vi "Calibrate_Axis_Sub.vi"(4 "Camera":T2="Pencilcam", 5 "Min Position":dbl=-1100.0, 6 "Position of Strip Centre":dbl=50.0, 7 "Max Position":dbl=1000.0, 8 "Time String":string, 9 "Axis to Calibrate":enum16{"X Axis", "Y Axis"}(ring), 10 "Datum Position":sgl[](array[numeric])=[0.0, 0.0, 50.0] format="%#.2f", 11 "Traverse Name":string="EnFlo_Stack") -> (0 "Status":T1, 1 "Correction Folder":path)   [LabVIEW 2015]
uses:
  Camera Server/Camera enum/Camera enum.ctl
  Multi_Run_Status.ctl
  Traverse_cluster.ctl
  Spacing.ctl
  Controls/Multi_run_mode.ctl
  Utilities/Image acquisition and processing/Feature detection/Typedefs/Top level controls.ctl
  Utilities/Image acquisition and processing/Feature detection/Typedefs/Theta range.ctl
  Utilities/Image acquisition and processing/Feature detection/Typedefs/Txy range.ctl
  Utilities/Image acquisition and processing/Feature detection/Typedefs/ROI bounds.ctl
  Camera Server/Camera enum/Camera resolution.ctl
  Controls/Tunnel_Coordinates.ctl
  Globals/Constants_global.vi
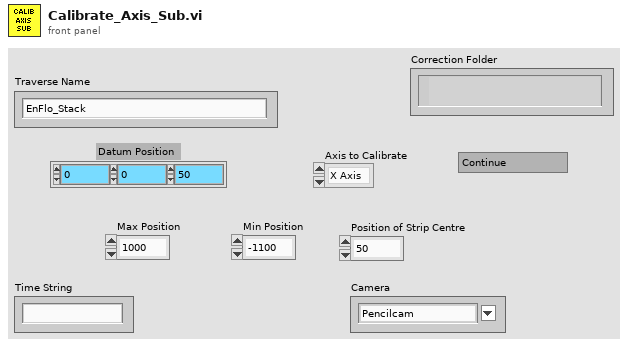
[diagram p1: front panel]
types:
  T1 = typedef "Multi_Run_Status.ctl" = enum16{"Continue", "Jump to Next Point", "Jump to Next Row", "Jump To Fall Back", "Terminate Run"}
  T2 = typedef "Camera enum.ctl" = string
  T3 = typedef "Traverse_cluster.ctl" = cluster{"Start X":sgl, "Start Y":sgl, "Start Z":sgl, "End X":sgl, "End Y":sgl, "End Z":sgl, "No. of pts.":i32, "Spacing":T4, "Filename":path, "Tunnel Speed":dbl, "Averaging time (min)":dbl, "Extra Commands":string, "Carrier_1 Q (l/min)":dbl, "Carrier_2 Q (l/min)":dbl, "Trace Gas Concentration (%)":dbl, "Specific Arguments":string, "Comments":string, "Row No":i32, "Row Type Selector":T5, "Completion time":string, "Row Duration (mins)":dbl, "No. of Valid pts.":i32, "Meas Setup File":string}
  T4 = typedef "Spacing.ctl" = enum16{"Linear", "Log", "Gauss", "Specified", "N/A"}
  T5 = typedef "Multi_run_mode.ctl" = enum16{"Move Traverse Only", "Set Tunnel Speed Only", "Set Source Only", "Set Measurement Conditions", "Single Measurement", "Vertical Profile", "Lateral Profile", "Longitudinal Profile", "Explore Volume", "Multi-Axis Profile", "Auto Calibrate", "Meas Fast FID Bkgnd", "Check Beam Power", "Scanning Valve Measurement", "Run VI Named:", "Set ADAM Ch", "Wait (minutes)", "Send Message", "Synchronize With:", "Fall Back to this Row", "Turn Off Row Repeating", "Blank Row", "Traverse 3D Volume"}
  T6 = typedef "ROI bounds.ctl" = cluster{"Xmax":i32, "Ymax":i32, "Xmin":i32, "Ymin":i32}
  T7 = typedef "Txy range.ctl" = cluster{"Tx max (pix)":i32, "Tx min (pix)":i32, "Ty max (pix)":i32, "Ty min (pix)":i32}
  T8 = typedef "Theta range.ctl" = cluster{"theta max (deg)":dbl, "theta min (deg)":dbl}
  T9 = typedef "Top level controls.ctl" = cluster{"Auto ROI (for rot.)":bool, "Apply scaling":bool, "Apply rotation":bool, "Apply Tx":bool, "Apply Ty":bool, "Keep proc. img":bool}
  T10 = enum16{"Load Command File", "Save Command File", "Check Multi Run Prog", "Check Multi Run Prog With Live Moves", "Run Multi Run Prog"}
  T11 = typedef "Tunnel_Coordinates.ctl" = enum16{"Work in Tunnel Coordinates", "Work in Model Coordinates"}
  T12 = typedef "Camera resolution.ctl" = u8
  T13 = enum16{"Load Command File", "Save Command File", "Check Multi Run Prog", "Check Multi Run Prog With Live Moves", "Run Multi Run Prog"}[]
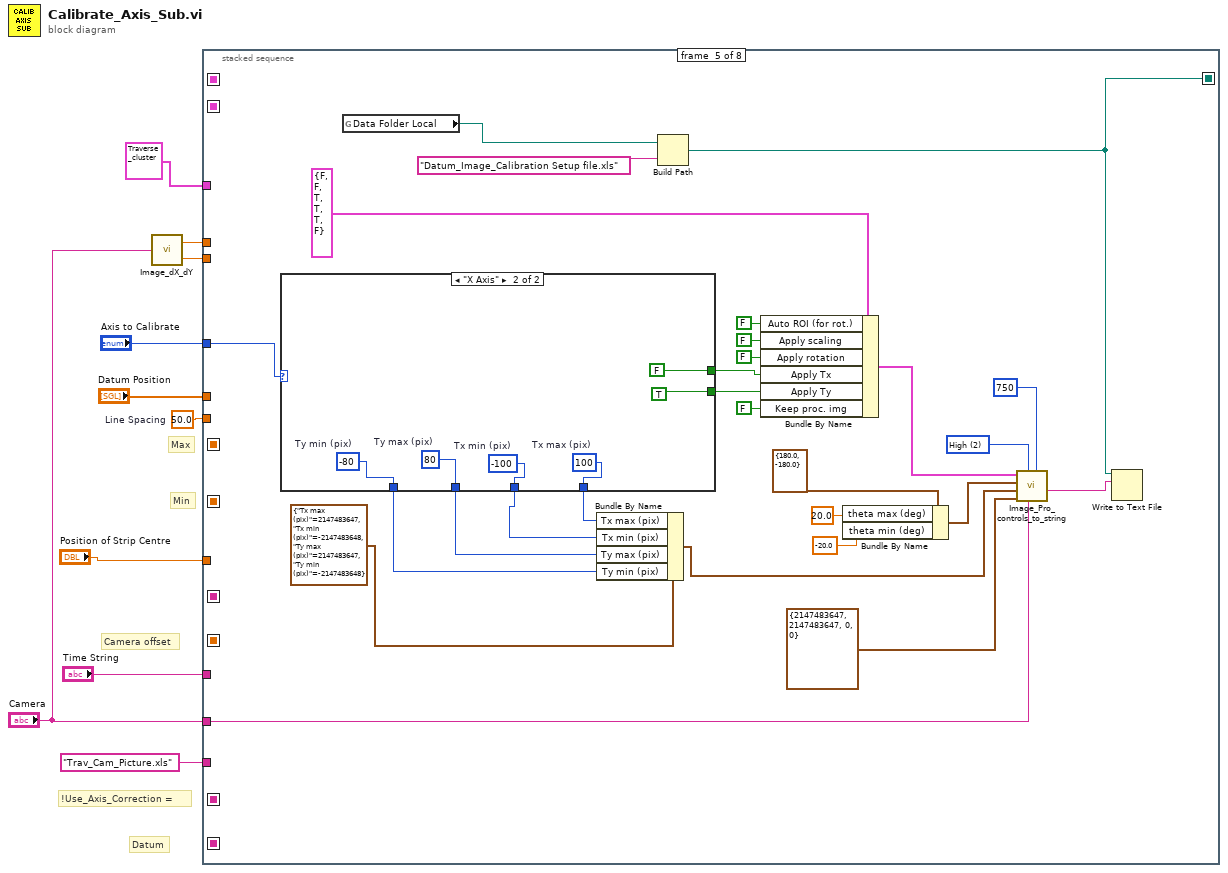
[diagram p0: block diagram]
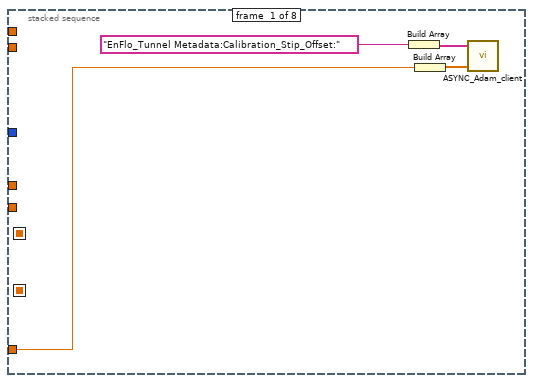
[diagram p2: hidden frame]
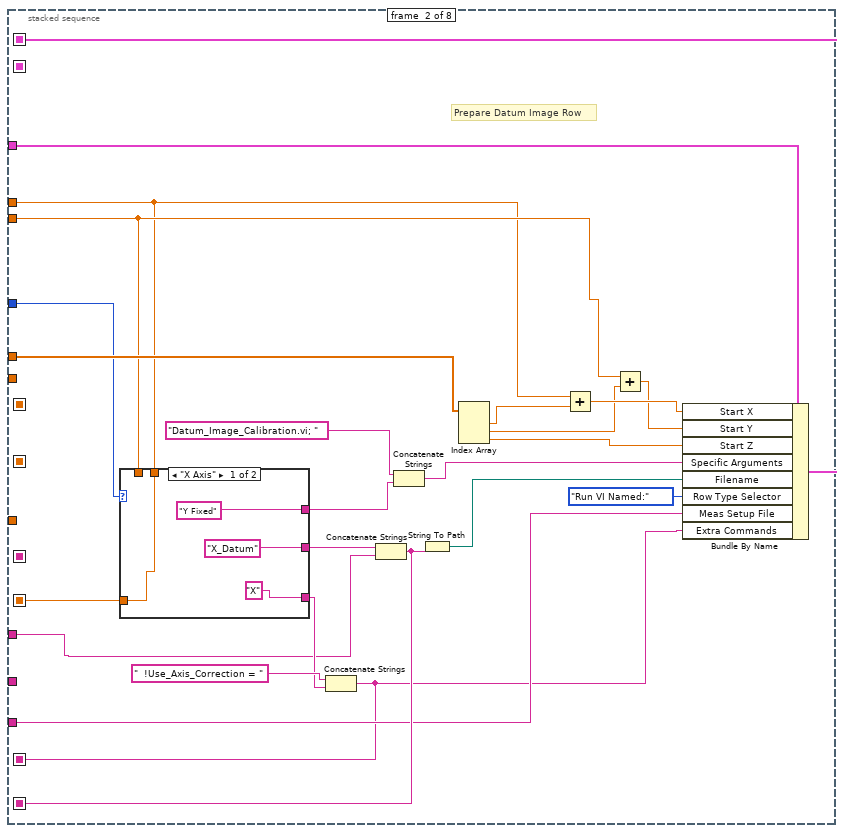
[diagram p3: hidden frame]
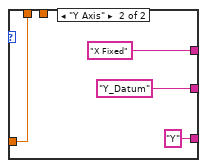
[diagram p4: hidden frame]
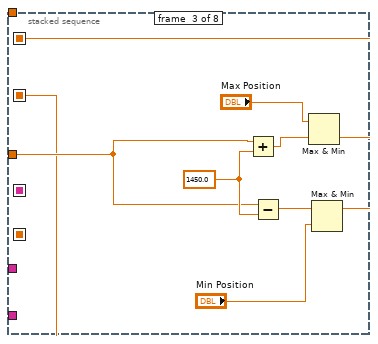
[diagram p5: hidden frame]
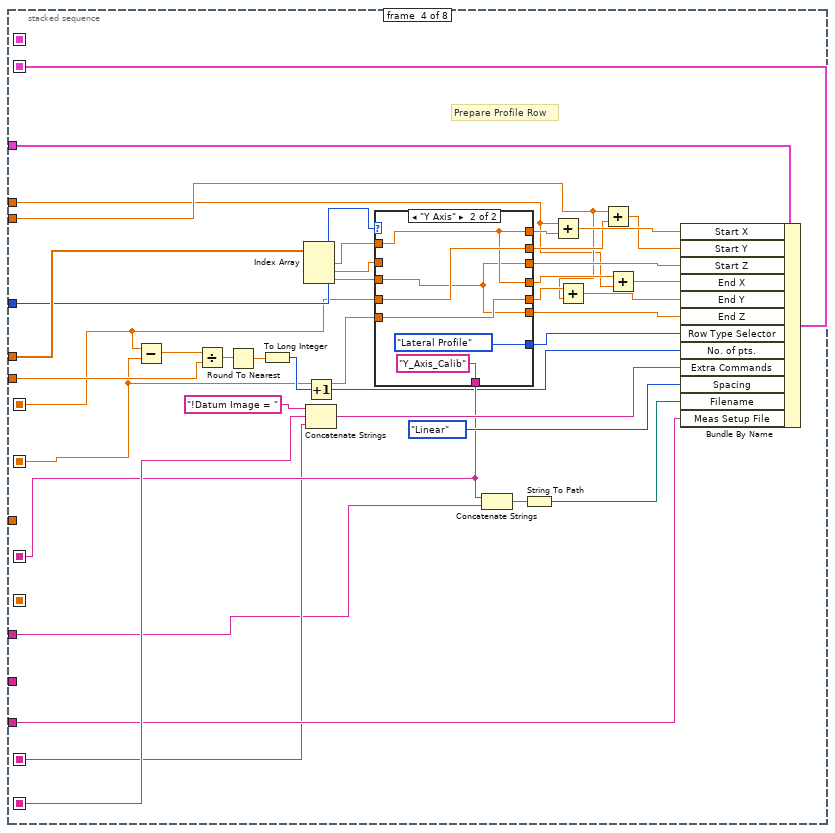
[diagram p6: hidden frame]
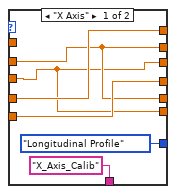
[diagram p7: hidden frame]
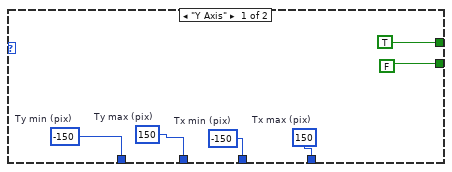
[diagram p8: hidden frame]
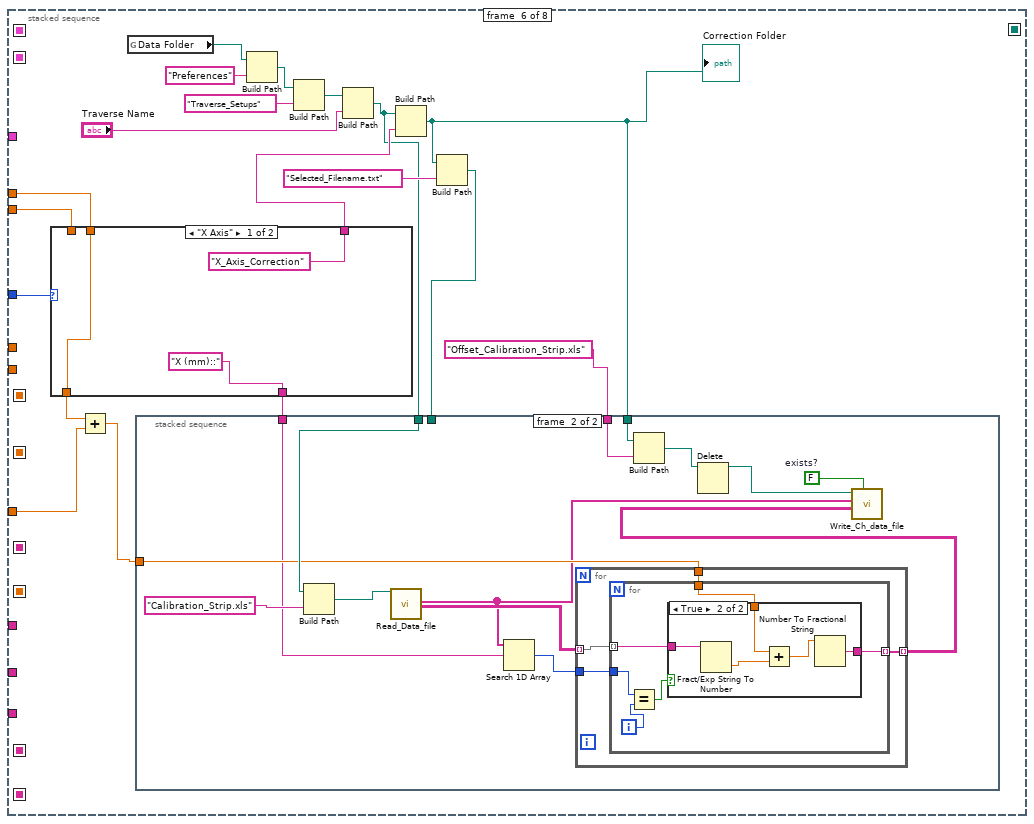
[diagram p9: hidden frame]
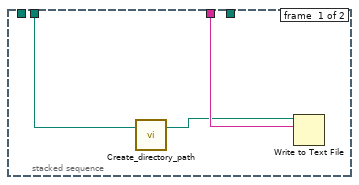
[diagram p10: hidden frame]
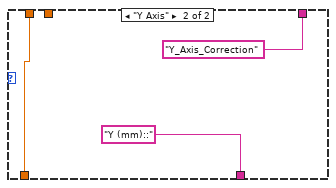
[diagram p12: hidden frame]
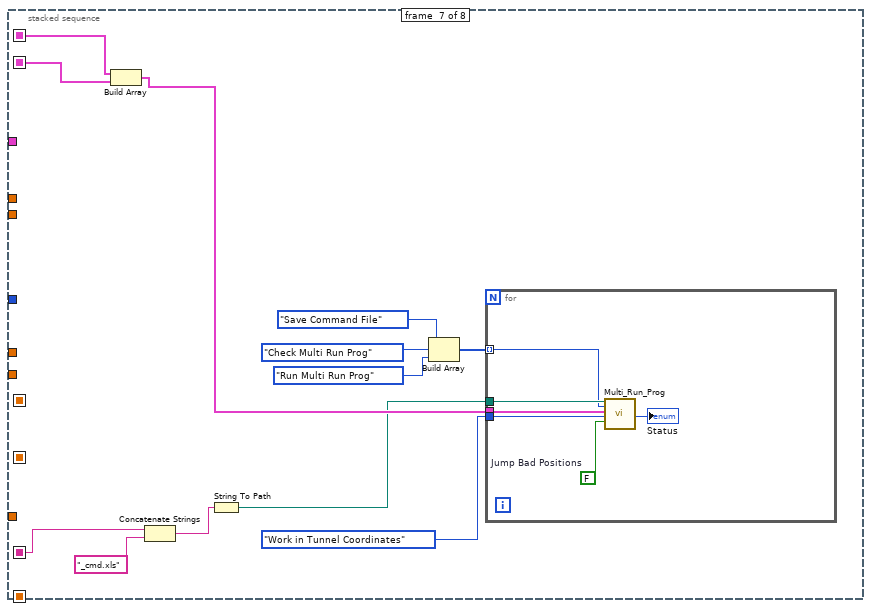
[diagram p13: hidden frame]
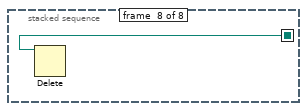
[diagram p14: hidden frame]
diagram:
  w5 = 50.0  # Line Spacing
  # "Camera offset"
  # "Min"
  # "Max"
  # "!Use_Axis_Correction ="
  # "Datum"
  n1 = call "Image_dX_dY.vi"("Camera"="Camera") -> ("X Offset"=w2:dbl, "Y Offset"=w1:dbl)
  n2 = stacked-sequence {
    seq-local: [_ w36 _ _ _ _ _ _] -> [_ _ _ _ _ _ w213 _]
    seq-local: [_ _ _ w77 _ _ _ _] -> [_ _ _ _ _ _ w212 _]
    seq-local: [_ w29 _ _ _ _ _ _] -> [_ _ _ w83 _ _ _ _]
    seq-local: [_ _ _ w71 _ _ _ _] -> [_ _ _ _ _ _ w210 _]
    seq-local: [_ _ _ _ w108 _ _ _] -> [_ _ _ _ _ _ _ w220]
    seq-local: [_ w23 _ _ _ _ _ _] -> [_ _ _ w69 _ _ _ _]
    seq-local: [_ _ w48 _ _ _ _ _] -> [_ _ _ w66 _ _ _ _]
    seq-local: [_ _ w47 _ _ _ _ _] -> [_ _ _ w65 _ _ _ _]
    seq-local: [_ w17 _ _ _ _ _ _] -> [_ _ _ _ _ _ _ _]
    tunnel: "Datum Position" -> [_ w38 _ w92 _ _ _ _]
    tunnel: "Axis to Calibrate" -> [_ w35 _ w91 w129 w155 _ _]
    tunnel: "Trav_Cam_Picture.xls" ("Meas Setup File") -> [_ w28 _ w73 _ _ _ _]
    tunnel: T3 {"Start X"=2010.0, "Start Y"=1100.0, "Start Z"=50.0, "End X"=2010.0, "End Y"=-1300.0, "End Z"=50.0, "No. of pts."=49, "Spacing"=enum."Linear", "Filename"=path "E:/Enflo_Data_Local/2016/EnFlo_Tunnel/Paul_Hayden/Results/Res_04-2016/Y_Axis_Calibration_Y+100.xls", "Tunnel Speed"=0.0, "Averaging time (min)"=0.05, "Extra Commands"="!Datum Image = 50mm_Y_Strip.xls", "Carrier_1 Q (l/min)"=0.0, "Carrier_2 Q (l/min)"=0.0, "Trace Gas Concentration (%)"=0.0, "Specific Arguments"="Y= ;1100 ; 1050 ; 1000 ; 950 ; 900 ; 850 ; 800 ; 750 ; 700 ; 650 ; 600 ; 550 ; 500 ; 450 ; 400 ; 350 ; 300 ; 250 ; 200 ; 150 ; 100 ; 50 ; 0 ; -50 ; -100 ; -150 ; -200 ; -250 ; -300 ; -350 ; -400 ; -450 ; -500 ; -550 ; -600 ; -650 ; -700 ; -750 ; -800 ; -850 ; -900 ; -950 ; -1000 ; -1050 ; -1100 ; -1150 ; -1200 ; -1250 ; -1300 ; ", "Comments"="", "Row No"=1, "Row Type Selector"=enum."Lateral Profile", "Completion time"="10:16  04-04-2016", "Row Duration (mins)"=10.616666666666667, "No. of Valid pts."=49, "Meas Setup File"="Trav_Cam_Picture.xls"} ("Traverse line") -> [_ w26 _ w72 _ _ _ _]
    tunnel: "Position of Strip Centre" -> [w11 _ w53 _ _ w145 _ _]
    tunnel: w5 -> [_ _ _ w68 _ _ _ _]
    tunnel: "Time String" -> [_ w22 _ w67 _ _ _ _]
    tunnel: "Camera" -> [_ _ _ _ w107 _ _ _]
    tunnel: w2 -> [_ w15 _ w57 _ w148 _ _]
    tunnel: w1 -> [_ w16 _ w58 _ w147 _ _]
    frame #0 {
      n3 = Build Array("EnFlo_Tunnel Metadata:Calibration_Stip_Offset:") -> (w13:string[])
      n4 = Build Array(w11) -> (w14:dbl[])
      n5 = call "ASYNC_Adam_client.vi"("Values"=w14, "Channel Names"=w13) -> ()  [unwired: 1 in, 2 out]
    }
    frame #1 {
      # "Prepare Datum Image Row"
      n6 = case shown="\"X Axis\"" w35 {
        tunnel: ["Y Fixed" "X Fixed"] -> w33
        tunnel: ["X_Datum" ("format string") "Y_Datum" ("format string")] -> w31
        tunnel: ["X" ("format string") "Y" ("format string")] -> w24
        tunnel: [w39 w43] -> w17
        tunnel: w16 -> [_ w43]
        tunnel: w15 -> [w39 _]
        frame "X Axis" {
        }
        frame "Y Axis" {
        }
      }
      n7 = Concatenate Strings("  !Use_Axis_Correction = ", w24) -> (w23:string)
      n8 = Concatenate Strings(w31, w22) -> (w29:string)
      n9 = Concatenate Strings("Datum_Image_Calibration.vi; " ("Specific Arguments"), w33) -> (w32:string)
      n10 = String To Path(string=w29) -> (path=w30:path)
      n11 = Index Array(array=w38) -> (element #1=w21:sgl, element #2=w19:sgl, element #3=w37:sgl)  [unwired: 3 in]
      n12 = Add(x=w15, y=w21) -> (x+y=w20:dbl)
      n13 = Add(x=w16, y=w19) -> (x+y=w18:dbl)
      n14 = Bundle By Name(cluster=w26, "Start X"=w20, "Start Y"=w18, "Start Z"=w37, "Specific Arguments"=w32, "Filename"=w30, "Row Type Selector"=Multi_run_mode."Run VI Named:", "Meas Setup File"=w28, "Extra Commands"=w23) -> (w36:T3)
    }
    frame #2 {
      w54 = 1450.0 ("y")
      n15 = Add(x=w53, y=w54) -> (x+y=w52:dbl)
      n16 = Subtract(x=w53, y=w54) -> (x-y=w50:dbl)
      n17 = Max & Min(x="Max Position", y=w52) -> (min(x,y)=w48:dbl)  [unwired: 1 out]
      n18 = Max & Min(x=w50, y="Min Position") -> (max(x,y)=w47:dbl)  [unwired: 1 out]
    }
    frame #3 {
      # "Prepare Profile Row"
      n19 = Subtract(x=w66, y=w65) -> (x-y=w82:dbl)
      n20 = Divide(x=w82, y=w68) -> (x/y=w81:dbl)
      n21 = Round To Nearest(number=w81) -> (nearest integer value=w80:dbl)
      n22 = To Long Integer(number=w80) -> (32bit integer=w79:i32)
      n23 = Index Array(array=w92) -> (element #1=w90:sgl, element #2=w86:sgl, element #3=w88:sgl)  [unwired: 3 in]
      n24 = Increment(x=w79) -> (x+1=w70:i32)
      n25 = Concatenate Strings("!Datum Image = " ("Extra Commands"), w83, w69) -> (w78:string)
      n26 = case shown="\"Y Axis\"" w91 {
        tunnel: [w96 w104] -> w62
        tunnel: w66 -> [w98 w104]
        tunnel: w65 -> [w97 w103]
        tunnel: [w96 w103] -> w59
        tunnel: w90 -> [_ w102]
        tunnel: [w98 w102] -> w64
        tunnel: [w95 w101] -> w89
        tunnel: w88 -> [w95 w101]
        tunnel: [w97 w102] -> w60
        tunnel: [w95 w101] -> w87
        tunnel: w86 -> [w96 _]
        tunnel: [Multi_run_mode."Longitudinal Profile" ("Row Type Selector") Multi_run_mode."Lateral Profile" ("Row Type Selector")] -> w85
        tunnel: ["X_Axis_Calib" ("format string") "Y_Axis_Calib" ("format string")] -> w71
        frame "X Axis" {
        }
        frame "Y Axis" {
        }
      }
      n27 = Concatenate Strings(w71, w67) -> (w75:string)
      n28 = String To Path(string=w75) -> (path=w74:path)
      n29 = Add(x=w57, y=w64) -> (x+y=w63:dbl)
      n30 = Add(x=w59, y=w58) -> (x+y=w55:dbl)
      n31 = Add(x=w58, y=w62) -> (x+y=w61:dbl)
      n32 = Add(x=w60, y=w57) -> (x+y=w56:dbl)
      n33 = Bundle By Name(cluster=w72, "Start X"=w63, "Start Y"=w61, "Start Z"=w89, "End X"=w56, "End Y"=w55, "End Z"=w87, "Row Type Selector"=w85, "No. of pts."=w70, "Extra Commands"=w78, "Spacing"=Spacing."Linear", "Filename"=w74, "Meas Setup File"=w73) -> (w77:T3)
    }
    frame #4 {
      w105 = T12 2 items=["Low", "Med.", "High", "Max."] ("Resolution")
      n34 = case shown="\"X Axis\"" w129 {
        tunnel: [FALSE ("Apply Ty") TRUE ("Apply Ty")] -> w123
        tunnel: [TRUE ("Apply Tx") FALSE ("Apply Tx")] -> w122
        tunnel: [w135 w141] -> w115
        tunnel: [w134 w140] -> w114
        tunnel: [w133 w139] -> w113
        tunnel: [w132 w138] -> w112
        frame "Y Axis" {
          w134 = -150  # Tx min (pix)
          w133 = 150  # Ty max (pix)
          w132 = -150  # Ty min (pix)
          w135 = 150  # Tx max (pix)
        }
        frame "X Axis" {
          w140 = -100  # Tx min (pix)
          w139 = 80  # Ty max (pix)
          w138 = -80  # Ty min (pix)
          w141 = 100  # Tx max (pix)
        }
      }
      n35 = global read "Constants_global.vi" "Data Folder Local"() -> (w130:path)
      n36 = Bundle By Name(cluster=T7 {"Tx max (pix)"=2147483647, "Tx min (pix)"=-2147483648, "Ty max (pix)"=2147483647, "Ty min (pix)"=-2147483648} ("Txy range (pixels)"), "Tx max (pix)"=w115, "Tx min (pix)"=w114, "Ty max (pix)"=w113, "Ty min (pix)"=w112) -> (w111:T7)
      n37 = Build Path(base path=w130, name or relative path="Datum_Image_Calibration Setup file.xls") -> (appended path=w108:path)
      n38 = Bundle By Name(cluster=T9 {"Auto ROI (for rot.)"=FALSE, "Apply scaling"=FALSE, "Apply rotation"=TRUE, "Apply Tx"=TRUE, "Apply Ty"=TRUE, "Keep proc. img"=FALSE} ("Controls"), "Auto ROI (for rot.)"=FALSE, "Apply scaling"=FALSE, "Apply rotation"=FALSE, "Apply Tx"=w122, "Apply Ty"=w123, "Keep proc. img"=FALSE) -> (w121:T9)
      n39 = Bundle By Name(cluster=T8 {"theta max (deg)"=180.0, "theta min (deg)"=-180.0} ("Theta range (deg)"), "theta max (deg)"=20.0, "theta min (deg)"=-20.0) -> (w119:T8)
      n40 = call "Image_Pro_controls_to_string.vi"("Quality"=u32 750, "Camera"=w107, "Resolution"=w105, "ROI to crop (pixels)"=T6 {"Xmax"=2147483647, "Ymax"=2147483647, "Xmin"=0, "Ymin"=0}, "Txy range (pixels)"=w111, "Theta range (deg)"=w119, "Controls"=w121) -> ("Setup String"=w109:string)  [unwired: 4 in]
      n41 = Write to Text File(file (use dialog)=w108, text=w109) -> ()  [unwired: 2 in, 3 out]
    }
    frame #5 {
      n42 = case shown="\"X Axis\"" w155 {
        tunnel: ["X_Axis_Correction" ("name or relative path") "Y_Axis_Correction" ("name or relative path")] -> w154
        tunnel: ["X (mm)::" ("String") "Y (mm)::" ("String")] -> w152
        tunnel: w148 -> [w196 _]
        tunnel: w147 -> [_ w199]
        tunnel: [w196 w199] -> w146
        frame "X Axis" {
        }
        frame "Y Axis" {
        }
      }
      n43 = Add(x=w146, y=w145) -> (x+y=w144:dbl)
      n44 = global read "Constants_global.vi" "Data Folder"() -> (w159:path)
      n45 = Build Path(base path=w159, name or relative path="Preferences") -> (appended path=w161:path)
      n46 = Build Path(base path=w161, name or relative path="Traverse_Setups") -> (appended path=w162:path)
      n47 = Build Path(base path=w162, name or relative path="Traverse Name") -> (appended path=w153:path)
      n48 = Build Path(base path=w153, name or relative path=w154) -> (appended path=w151:path)
      "Correction Folder" <- w151
      n49 = Build Path(base path=w151, name or relative path="Selected_Filename.txt" ("Substring")) -> (appended path=w149:path)
      n50 = stacked-sequence {
        tunnel: w153 -> [_ w179]
        tunnel: w144 -> [_ w174]
        tunnel: w152 -> [_ w173]
        tunnel: w151 -> [_ w170]
        tunnel: "Offset_Calibration_Strip.xls" ("name or relative path") -> [w164 w169]
        tunnel: w149 -> [w165 _]
        frame #0 {
          n51 = call "Create_directory_path.vi"("Path name"=w165) -> ("Path name Out"=w163:path)  [unwired: 1 in, 1 out]
          n52 = Write to Text File(file (use dialog)=w163, text=w164) -> ()  [unwired: 2 in, 3 out]
        }
        frame #1 {
          w172 = FALSE  # exists?
          n53 = Build Path(base path=w179, name or relative path="Calibration_Strip.xls") -> (appended path=w177:path)
          n54 = call "Read_Data_file.vi"("Results file"=w177) -> ("Ch names Out"=w171:string[], "Channel Values Out"=w175:string[][])  [unwired: 4 in, 13 out]
          n55 = Search 1D Array(1D array=w171, element=w173) -> (index of element=w176:i32)  [unwired: 1 in]
          n56 = for {
            tunnel: w176 -> [w181]
            tunnel: w175 -> [w182] mode=indexing
            tunnel: w174 -> [w183]
            tunnel: [w180] -> w168 mode=indexing
            n57 = for {
              tunnel: w183 -> [w189]
              tunnel: w182 -> [w188] mode=indexing
              tunnel: w181 -> [w187]
              tunnel: [w184] -> w180 mode=indexing
              i -> [w186]
              n58 = Equal?(x=w187, y=w186) -> (x = y?=w185:bool)
              n59 = case shown="True" w185 {
                tunnel: w189 -> [_ w194]
                tunnel: w188 -> [w190 w192]
                tunnel: [w190 w191] -> w184
                frame False {
                }
                frame True {
                  n60 = Fract/Exp String To Number(string=w192) -> (number=w195:dbl)  [unwired: 3 in, 1 out]
                  n61 = Add(x=w194, y=w195) -> (x+y=w193:dbl)
                  n62 = Number To Fractional String(number=w193) -> (F-format string=w191:string)  [unwired: 3 in]
                }
              }
            }
          }
          n63 = Build Path(base path=w170, name or relative path=w169) -> (appended path=w167:path)
          n64 = Delete(path (use dialog)=w167) -> (deleted path=w166:path)  [unwired: 4 in, 2 out]
          n65 = call "Write_Ch_data_file.vi"("exists?"=w172, "Channel Values"=w168, "Channel names"=w171, "Filename"=w166) -> ()  [unwired: 3 in, 5 out]
        }
      }
    }
    frame #6 {
      n66 = Build Array(w213, w212) -> (w211:T3[])
      n67 = Concatenate Strings(w210, "_cmd.xls" ("string")) -> (w207:string)
      n68 = String To Path(string=w207) -> (path=w208:path)
      n69 = Build Array(T10."Save Command File" ("Mode"), T10."Check Multi Run Prog" ("Mode"), T10."Run Multi Run Prog" ("Mode")) -> (w202:T13)
      n70 = for {
        tunnel: w211 -> [w219]
        tunnel: w208 -> [w218]
        tunnel: Tunnel_Coordinates."Work in Tunnel Coordinates" ("Work in Tunnel Coordinates?") -> [w217]
        tunnel: w202 -> [w216] mode=indexing
        w215 = FALSE  # Jump Bad Positions
        n71 = call "Multi_Run_Prog.vi"("Command filename"=w218, "Mode"=w216, "Table"=w219, "Work in Tunnel Coordinates?"=w217, "Jump Bad Positions"=w215) -> ("Status"=→"Status":T1)  [unwired: 14 in]
      }
    }
    frame #7 {
      n72 = Delete(path (use dialog)=w220) -> ()  [unwired: 4 in, 3 out]
    }
  }
